vi "Edit Tree Items-Add Item.vi"(4 "Child Only?":bool, 5 "Child Tag":string, 6 "Child Text":string[](array[string]), 7 "Left Cell String":string, 8 "error in (no error)":errorcluster, 9 "Child Position":i32, 10 "Parent Tag":string, 11 "TreeControl in":refnum<class "TreeControl.lvclass">) -> (0 "error out":errorcluster, 2 "Edit Tree Items:Add Item":string, 3 "TreeControl out":refnum<class "TreeControl.lvclass">)   [LabVIEW 2015, in "TreeControl.lvclass"]
doc: "Adds an item to the tree control.\n\n This method is similar to the <b>Insert Item Before</b> item on the shortcut menu of a tree control.\n\nQControl Class wrapper around the <b>TreeControl : Edit Tree Items:Add Item Method</b>.\n<b> </b> <b> </b>\n©2016 Q Software Innovations, LLC (QSI)\nwritten by Quentin Alldredge\nproduced in LabVIEW 2015\n\nsupport@qsoftwareinnovations.com\nwww.qsoftwareinnovations.com\n\nAll rights reserved.\n\nRedistribution and use in source and binary forms, with or without modification, are permitted provided that the following conditions are met:\n\n * Redistributions of source code must retain the above copyright notice, this list of conditions and the following disclaimer.\n * Redistributions in binary form must reproduce the above copyright notice, this list of conditions and the following disclaimer in the documentation and/or other materials provided with the distribution.\n * Neither the name of Q Software Innovations, LLC. nor the names of its contributors may be used to endorse or promote products derived from this software without specific prior written permission.\n\nTHIS SOFTWARE IS PROVIDED BY THE COPYRIGHT HOLDERS AND CONTRIBUTORS \"AS IS\" AND ANY EXPRESS OR IMPLIED WARRANTIES, INCLUDING, BUT NOT LIMITED TO, THE IMPLIED WARRANTIES OF MERCHANTABILITY AND FITNESS FOR A PARTICULAR PURPOSE ARE DISCLAIMED. IN NO EVENT SHALL THE COPYRIGHT OWNER OR CONTRIBUTORS BE LIABLE FOR ANY DIRECT, INDIRECT, INCIDENTAL, SPECIAL, EXEMPLARY, OR CONSEQUENTIAL DAMAGES (INCLUDING, BUT NOT LIMITED TO, PROCUREMENT OF SUBSTITUTE GOODS OR SERVICES; LOSS OF USE, DATA, OR PROFITS; OR BUSINESS INTERRUPTION) HOWEVER CAUSED AND ON ANY THEORY OF LIABILITY, WHETHER IN CONTRACT, STRICT LIABILITY, OR TORT (INCLUDING NEGLIGENCE OR OTHERWISE) ARISING IN ANY WAY OUT OF THE USE OF THIS SOFTWARE, EVEN IF ADVISED OF THE POSSIBILITY OF SUCH DAMAGE."
uses:
  TreeControl.lvclass
  TreeControl.lvclass/TreeControl.ctl
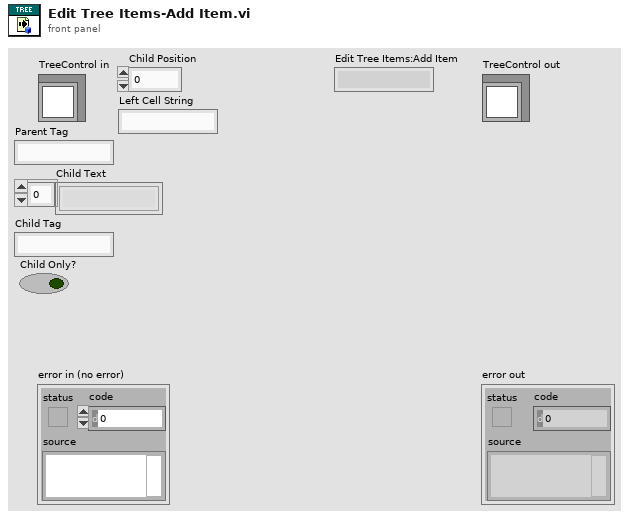
[diagram p1: front panel]
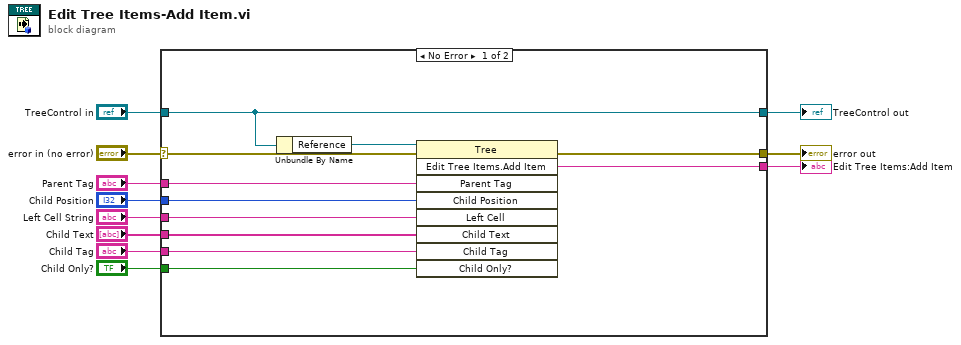
[diagram p0: block diagram]
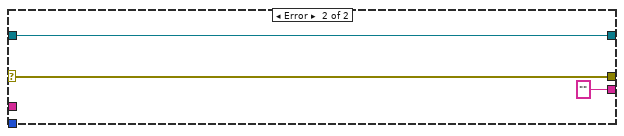
[diagram p2: hidden frame]
diagram:
  n1 = case shown="No Error" "error in (no error)" {
    selector: "error in (no error)" -> [w22 w25]
    tunnel: [w21 w25] -> w10
    tunnel: [w20 w24] -> w8
    tunnel: "TreeControl in" -> [w20 w24]
    tunnel: "Parent Tag" -> [w18 _]
    tunnel: [w17 "" ("Edit Tree Items:Add Item")] -> w6
    tunnel: "Child Position" -> [w16 _]
    tunnel: "Left Cell String" -> [w15 _]
    tunnel: "Child Text" -> [w14 _]
    tunnel: "Child Tag" -> [w13 _]
    tunnel: "Child Only?" -> [w12 _]
    frame No Error {
      n2 = Unbundle By Name(w20) -> ("Reference"=w19:refnum<vi>)
      n3 = invoke class="Tree" method="Edit Tree Items.Add Item"(reference=w19, error in=w22, "Parent Tag"=w18, "Child Position"=w16, "Left Cell"=w15, "Child Text"=w14, "Child Tag"=w13, "Child Only?"=w12) -> (error out=w21:errorcluster, "Edit Tree Items:Add Item"=w17:string)  [unwired: 1 in, 7 out]
    }
    frame Error {
    }
  }
  "error out" <- w10
  "TreeControl out" <- w8
  "Edit Tree Items:Add Item" <- w6
